vi "测试VI专用.vi"() -> ()   [LabVIEW 2013]
panel:
  out "数值":dbl
  in  "停止":bool
  out "数组 3":i32[](array[numeric])
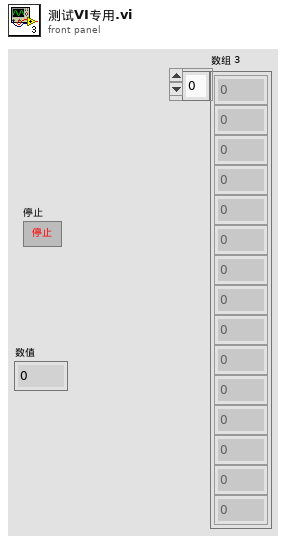
[diagram p1: front panel]
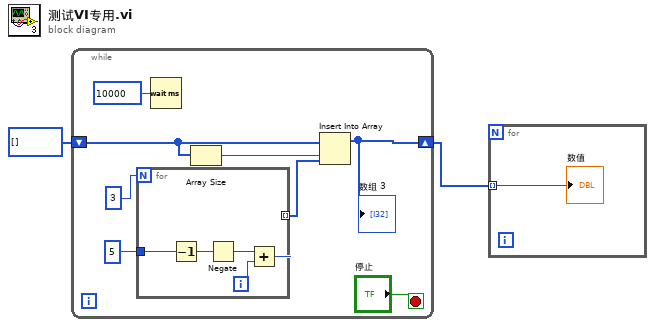
[diagram p0: block diagram]
diagram:
  n1 = while {
    shift-right: [w3] -> w1
    shift-left: i32[] [] -> [w7]
    stop <- "停止" stop-if-true
    n2 = for {
      N: 3 -> [_]
      tunnel: 5 -> [w12]
      tunnel: [w11] -> w8 mode=indexing
      i -> [w13]
      n3 = Decrement(x=w12) -> (x-1=w15:i32)
      n4 = Negate(x=w15) -> (-x=w14:i32)
      n5 = Add(x=w14, y=w13) -> (x+y=w11:i32)
    }
    n6 = Wait (ms)(milliseconds to wait=u32 10000 ("等待时间（毫秒）")) -> ()  [unwired: 1 out]
    n7 = Array Size(array=w7) -> (size(s)=w6:i32)
    n8 = Insert Into Array(array=w7, index=w6, new element=w8) -> (w3:i32[])
    "数组 3" <- w3
  }
  n9 = for {
    tunnel: w1 -> [w16] mode=indexing
    "数值" <- w16
  }
